vi "Client TCP Request PDF Print.vi"(8 "error in (no error)":errorcluster, 10 "Client (\"\": localhost)":string, 11 "Report PDF Path":path) -> (0 "error out":errorcluster)   [LabVIEW 2011]
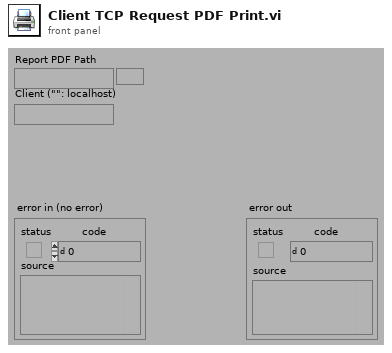
[diagram p1: front panel]
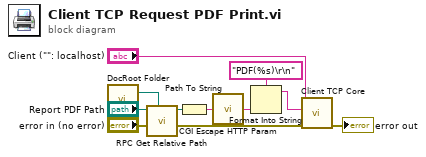
[diagram p0: block diagram]
diagram:
  n1 = call "DocRoot Folder.vi"() -> ("DocumentRoot Folder"=w1:path)  [unwired: 3 in]
  n2 = call "RPC Get Relative Path.vi"("Base Path (empty)"=w1, "Absolute Path (empty)"="Report PDF Path") -> ("Path Relative to Base"=w4:path)  [unwired: 3 out]
  n3 = Path To String(path=w4) -> (string=w3:string)
  n4 = call "CGI Escape HTTP Param.vi"("string"=w3) -> ("url-encoded string"=w2:string)
  n5 = Format Into String(format string="PDF(%s)\r\n", w2) -> (resulting string=w6:string)  [unwired: 2 in, 1 out]
  n6 = call "Client TCP Core.vi"("error in (no error)"="error in (no error)", "Command(Params) (\"\")"=w6, "Client (\"\": localhost)"="Client (\"\": localhost)") -> ("error out"=→"error out":errorcluster)  [unwired: 8 out]
